vi "Read From MFC.vi"(8 "error in (no error)":errorcluster, 10 "Device ID":string, 11 "VISA Sesssion In":refnum<visa-resource-name>="ASRL13::INSTR") -> (0 "error out":errorcluster, 2 "Output":string[](array[string]), 3 "VISA Sesssion Out":refnum<visa-resource-name>="ASRL6::INSTR")   [LabVIEW 2019]
uses:
  <vilib>/Instr/_visa.llb/VISA Flush IO Buffer Mask.ctl
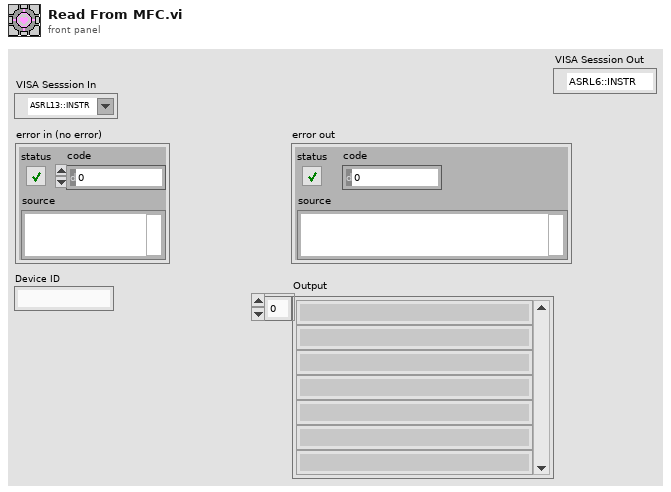
[diagram p1: front panel]
types:
  T1 = typedef "VISA Flush IO Buffer Mask.ctl" = u16
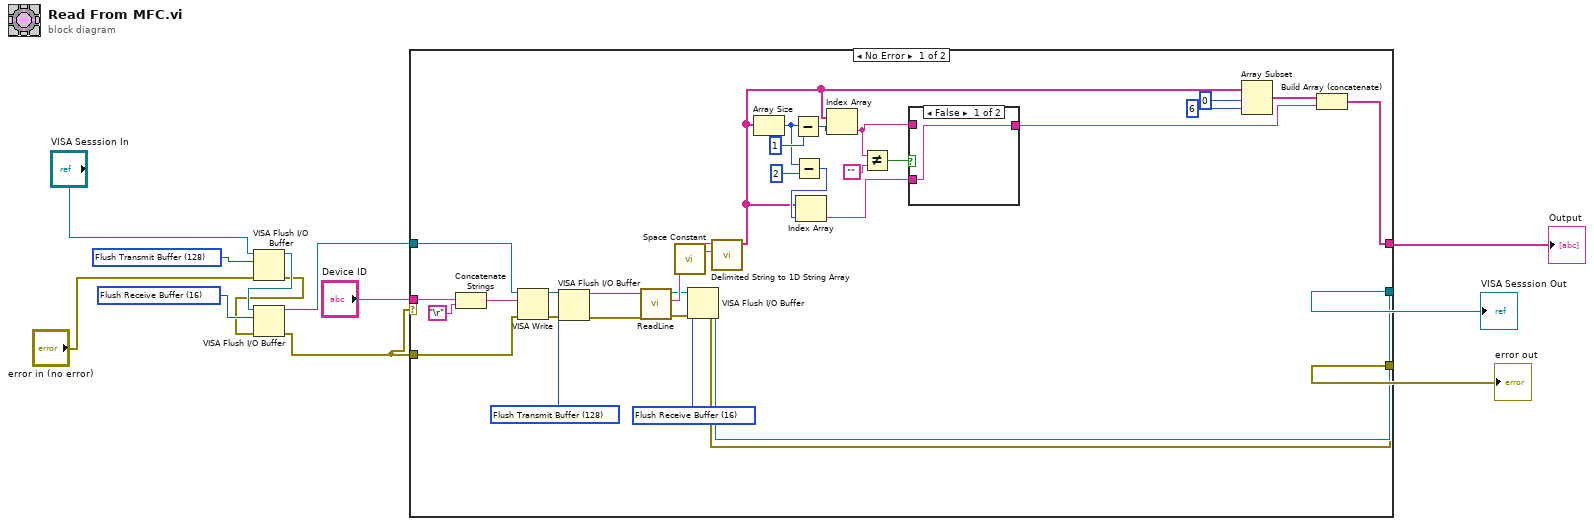
[diagram p0: block diagram]
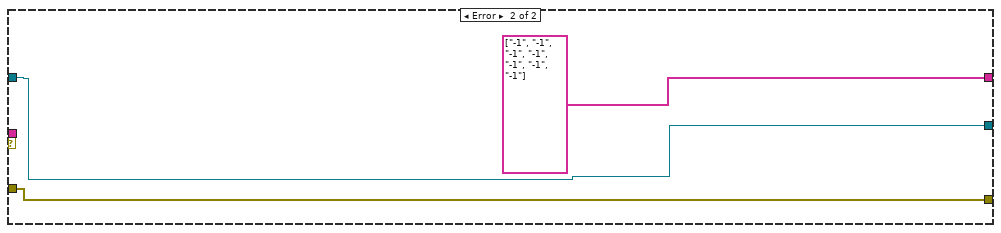
[diagram p3: hidden frame]
diagram:
  w7 = T1 16 items=["Flush Receive Buffer"=16, "Write Transmit Buffer to Device"=32, "Flush Receive Buffer (No I/O)"=64, "Flush Transmit Buffer"=128] ("Mask")
  w8 = T1 128 items=["Flush Receive Buffer"=16, "Write Transmit Buffer to Device"=32, "Flush Receive Buffer (No I/O)"=64, "Flush Transmit Buffer"=128] ("Mask")
  n1 = VISA Flush I/O Buffer(VISA resource name="VISA Sesssion In", mask (16)=w8, error in (no error)="error in (no error)") -> (VISA resource name out=w5:refnum<visa-resource-name>, error out=w2:errorcluster)
  n2 = VISA Flush I/O Buffer(VISA resource name=w5, mask (16)=w7, error in (no error)=w2) -> (VISA resource name out=w4:refnum<visa-resource-name>, error out=w1:errorcluster)
  n3 = case shown="No Error" w1 {
    tunnel: "Device ID" -> [w44 _]
    tunnel: [w41 w47] -> w10
    tunnel: w1 -> [w39 w49]
    tunnel: [w38 w49] -> w11
    tunnel: [w25 string[] ["-1", "-1", "-1", "-1", "-1", "-1", "-1"] ("string array")] -> w9
    tunnel: w4 -> [w28 w47]
    frame No Error {
      w34 = T1 16 items=["Flush Receive Buffer"=16, "Write Transmit Buffer to Device"=32, "Flush Receive Buffer (No I/O)"=64, "Flush Transmit Buffer"=128] ("Mask")
      w35 = T1 128 items=["Flush Receive Buffer"=16, "Write Transmit Buffer to Device"=32, "Flush Receive Buffer (No I/O)"=64, "Flush Transmit Buffer"=128] ("Mask")
      n4 = Concatenate Strings(w44, "\r") -> (w43:string)
      n5 = VISA Write(VISA resource name=w28, write buffer=w43, error in (no error)=w39) -> (VISA resource name out=w36:refnum<visa-resource-name>, error out=w37:errorcluster)  [unwired: 1 out]
      n6 = VISA Flush I/O Buffer(VISA resource name=w36, mask (16)=w35, error in (no error)=w37) -> (VISA resource name out=w33:refnum<visa-resource-name>, error out=w32:errorcluster)
      n7 = call "ReadLine.vi"("error in (no error)"=w32, "VISA Sesssion In"=w33) -> ("error out"=w29:errorcluster, "Read Line"=w31:string, "VISA Sesssion Out"=w30:refnum<visa-resource-name>)  [unwired: 7 in]
      n8 = call <vilib>:"Space Constant.vi"() -> ("String"=w42:string)
      n9 = VISA Flush I/O Buffer(VISA resource name=w30, mask (16)=w34, error in (no error)=w29) -> (VISA resource name out=w41:refnum<visa-resource-name>, error out=w38:errorcluster)
      n10 = call <vilib>:"Delimited String to 1D String Array.vi"("delimiter"=w42, "delimited string"=w31) -> ("string array"=w15:string[])  [unwired: 9 in]
      n11 = Array Size(array=w15) -> (size(s)=w18:i32)
      n12 = Subtract(x=w18, y=1) -> (x-y=w22:i32)
      n13 = Subtract(x=w18, y=2) -> (x-y=w16:i32)
      n14 = Index Array(array=w15, index=w16) -> (element=w14:string)
      n15 = Index Array(array=w15, index=w22) -> (element=w19:string)
      n16 = Not Equal?(x=w19, y="") -> (x != y?=w20:bool)
      n17 = case shown="False" w20 {
        tunnel: w19 -> [_ w46]
        tunnel: [w45 w46] -> w13
        tunnel: w14 -> [w45 _]
        frame False {
        }
        frame True {
        }
      }
      n18 = Array Subset(array=w15, index=0, length=6) -> (w24:string[])
      n19 = Build Array (concatenate)(w24, w13) -> (w25:string[])
    }
    frame Error {
    }
  }
  "Output" <- w9
  "error out" <- w11
  "VISA Sesssion Out" <- w10
